vi "Practica 4 itiw31.vi"() -> ()   [LabVIEW 2018]
uses:
  <vilib>/express/express analysis/Spectral/Block/exnSpectralBlock spectral measurements RMS poly.vi
  <vilib>/express/express analysis/Spectral/Block/exnSpectralBlock spectral measurements RMS DDT.vi
  <vilib>/express/express analysis/Spectral/XNode/ExpressSpectralMeasurementsBlockNode.xnode
panel:
  out "Graficas en el dominio de la frecuencia":dynamicdata(graph)
  out "Graficas de senal 1 y 2":dynamicdata(graph)
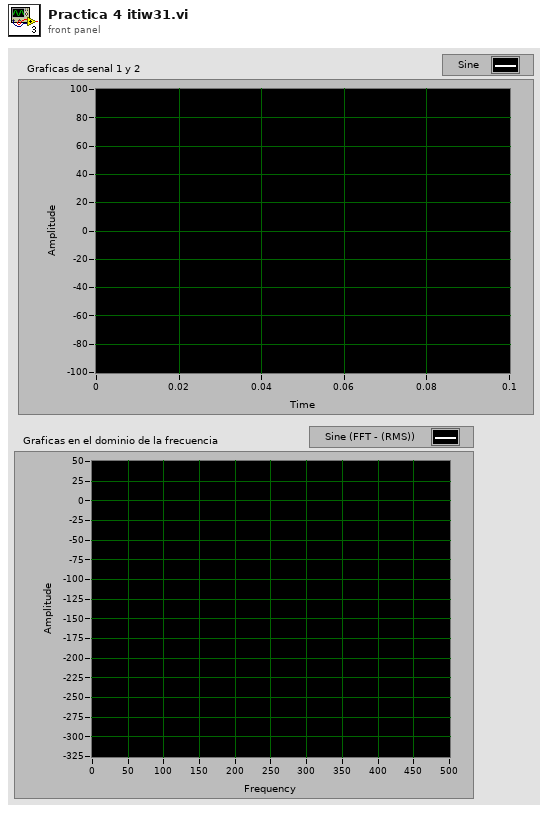
[diagram p1: front panel]
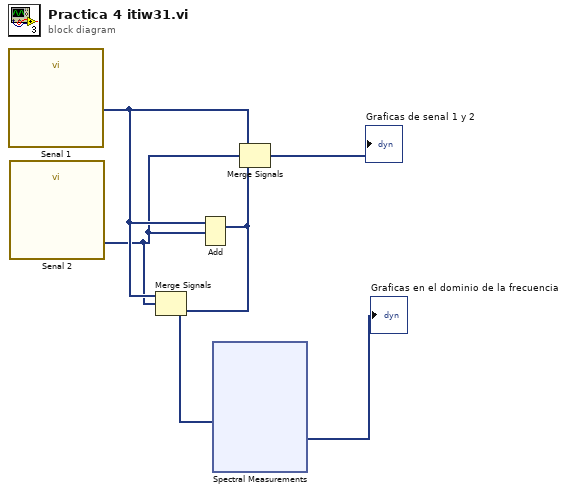
[diagram p0: block diagram]
diagram:
  n1 = call "Senal 1"() -> ("Sine"=w4:dynamicdata)  [unwired: 14 in, 1 out]
  n2 = call "Senal 2"() -> ("Sine"=w3:dynamicdata)  [unwired: 14 in, 1 out]
  n3 = Add(1:w3, 2:w4) -> (0:w2:dynamicdata)  [unwired: 1 in, 1 out]
  n4 = Merge Signals(w4, w3, w2) -> (w1:dynamicdata)
  n5 = xnode "Spectral Measurements"("Signals"=w1) -> ("FFT - (RMS)"=→"Graficas en el dominio de la frecuencia":dynamicdata)  [unwired: 1 in, 2 out]
  n6 = Merge Signals(w4, w3, w2) -> (→"Graficas de senal 1 y 2":dynamicdata)
